vi "Save.vi"(7 "source paths":path[](array[path]), 8 "error in":errorcluster, 10 "processed sources":refnum<class "AB_Source.lvclass">[](array[class]), 11 "AB_Build in":refnum<class "AB_Build.lvclass">) -> (0 "error out":errorcluster, 1 "TypeInfo":string, 2 "source destination paths":path[](array[path]), 3 "AB_Build out":refnum<class "AB_Build.lvclass">, 4 "eng_LEIFBuildData":u32, 5 "checksums":string[](array[string]))   [LabVIEW 2020, in "AB_Build.lvclass"]
uses:
  <vilib>/AppBuilder/AB_Classes/Build/AB_Build.lvclass
  <vilib>/AppBuilder/AB_Classes/Source/AB_Source.lvclass
  <vilib>/AppBuilder/AB_Classes/Build/AB_Build.lvclass/AB_Build.ctl
  <vilib>/AppBuilder/AB_Classes/Source/VI/AB_Source_VI.lvclass
  <resource>/Framework/Providers/Common/provcom_StringGlobals.vi
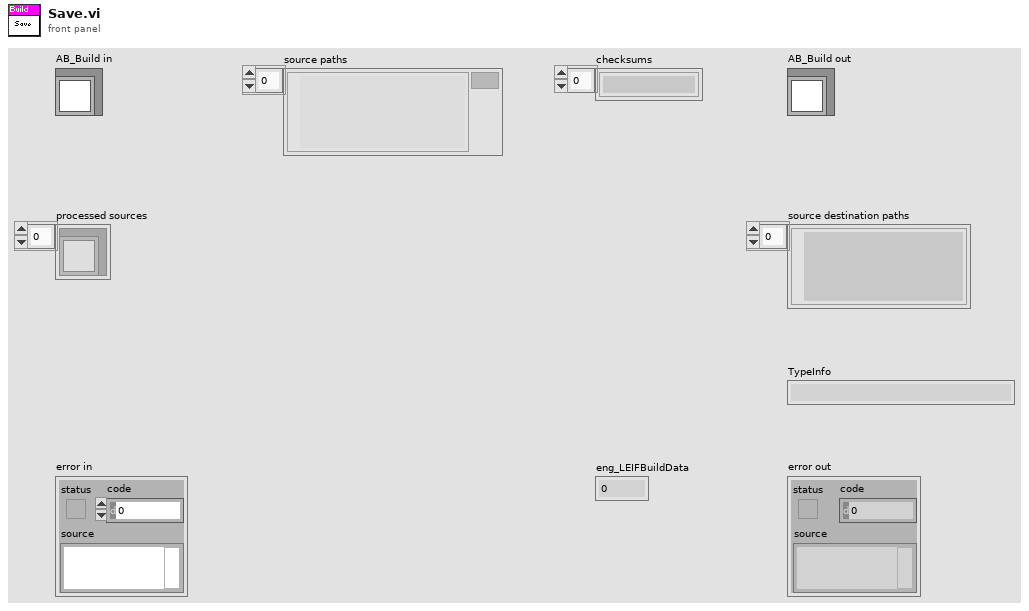
[diagram p1: front panel]
types:
  T1 = typedef "provcom_ProgressBar_Events.ctl" = cluster{"newJob":refnum<user-event>, "newItem":refnum<user-event>, "errorMsg":T2, "cancel":refnum<user-event>}
  T2 = typedef "mxLvBuildError.ctl" = refnum<user-event>
  T3 = typedef "AB_Source_Processed_Info.ctl" = cluster{"destPath":path, "buildDelimitedName":string, "sourceIndex":i32, "topLevel":bool}
  T4 = typedef "AB_Source_VI.ctl" = cluster{"standardVI":bool, "dynamicDispatch":bool, "LLBtopLevel":bool, "privateDataControl":bool, "eng_hasNonVILinks":bool, "eng_reference":refnum<vi>, "eng_saveLevel":u32}
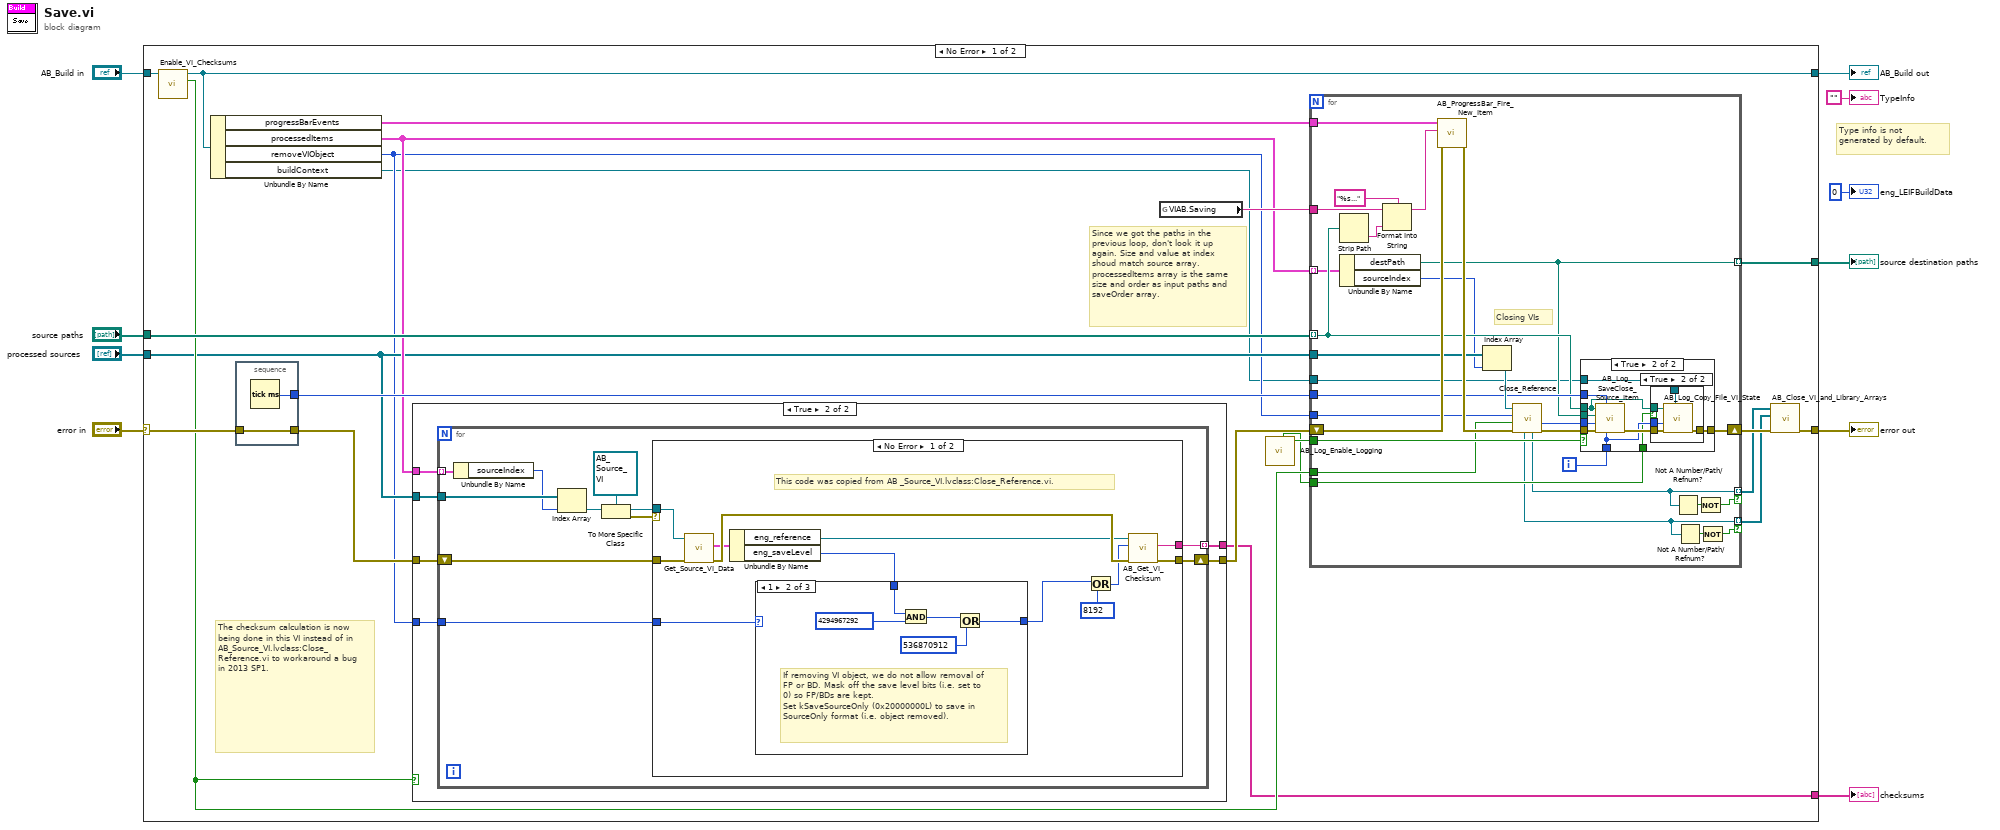
[diagram p0: block diagram]
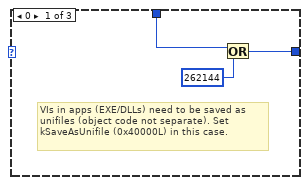
[diagram p3: hidden frame]
diagram:
  # "Type info is not generated by default."
  n1 = case shown="No Error" "error in" {
    selector: "error in" -> [w32 w122]
    tunnel: [w28 w122] -> w9
    tunnel: [w20 w121] -> w7
    tunnel: "AB_Build in" -> [w21 w121]
    tunnel: [w24 _] -> w6
    tunnel: "source paths" -> [w23 _]
    tunnel: "processed sources" -> [w17 _]
    tunnel: [w15 _] -> w2
    frame No Error {
      # "The checksum calculation is now being done in this VI instead of in AB_Source_VI.lvclass:Close_Reference.vi to workaround a bug in 2013 SP1."
      # "Since we got the paths in the previous loop, don't look it up again. Size and value at index shoud match source array. processedItems array is the same size and order as input paths and saveOrder array."
      n2 = call-dynamic "Enable_VI_Checksums.vi"("AB_Build in"=w21) -> ("VI checksums enabled?"=w19:bool, "AB_Build out"=w20:refnum<class "AB_Build.lvclass">)  [unwired: 8 in, 1 out]
      n3 = Unbundle By Name(w20) -> ("progressBarEvents"=w26:T1, "processedItems"=w18:T3[], "removeVIObject"=w16:u16, "buildContext"=w13:refnum<vi>)
      n4 = stacked-sequence {
        tunnel: w32 -> [w74]
        tunnel: [w74] -> w31
        tunnel: [w73] -> w22
        frame #0 {
          n5 = Tick Count (ms)() -> (millisecond timer value=w73:u32)
        }
      }
      n6 = case shown="True" w19 {
        tunnel: w31 -> [w33 w39]
        tunnel: [w33 w38] -> w30
        tunnel: w18 -> [_ w37]
        tunnel: w17 -> [_ w36]
        tunnel: [_ w35] -> w15
        tunnel: w16 -> [_ w34]
        frame False {
          # "Don't calculate checksums."
        }
        frame True {
          n7 = for {
            shift-right: [w48] -> w38
            shift-left: w39 -> [w49]
            tunnel: w37 -> [w47] mode=indexing
            tunnel: w36 -> [w46]
            tunnel: [w41] -> w35 mode=indexing
            tunnel: w34 -> [w40]
            n8 = Unbundle By Name(w47) -> ("sourceIndex"=w45:i32)
            n9 = Index Array(array=w46, index=w45) -> (element=w44:refnum<class "AB_Source.lvclass">)
            n10 = To More Specific Class(target class=refnum<class "AB_Source_VI.lvclass"> refnum ("AB_Source_VI.lvclass"), reference=w44) -> (specific class reference=w42:refnum<class "AB_Source_VI.lvclass">, error out=w50:errorcluster)  [unwired: 1 in]
            n11 = case shown="No Error" w50 {
              tunnel: w42 -> [w59 _]
              tunnel: w49 -> [w62 w72]
              tunnel: [w61 w72] -> w48
              tunnel: [w52 _] -> w41
              tunnel: w40 -> [w51 _]
              frame No Error {
                # "This code was copied from AB _Source_VI.lvclass:Close_Reference.vi."
                n12 = call <vilib>:"Get_Source_VI_Data.vi"("error in (no error)"=w62, "Class in"=w59) -> ("error out"=w60:errorcluster, "data"=w58:T4)  [unwired: 7 in, 1 out]
                n13 = Unbundle By Name(w58) -> ("eng_reference"=w57:refnum<vi>, "eng_saveLevel"=w54:u32)
                n14 = case shown="1" w51 {
                  tunnel: w54 -> [w65 w70 w71]
                  tunnel: [w64 w67 w71] -> w53
                  frame 0 {
                    # "VIs in apps (EXE/DLLs) need to be saved as unifiles (object code not separate). Set kSaveAsUnifile (0x40000L) in this case."
                    n15 = Or(x=w65, y=u32 262144 ("data.eng_saveLevel")) -> (x .or. y?=w64:u32)
                  }
                  frame 1 {
                    # "If removing VI object, we do not allow removal of FP or BD. Mask off the save level bits (i.e. set to 0) so FP/BDs are kept.\nSet kSaveSourceOnly (0x20000000L) to save in SourceOnly format (i.e. object removed)."
                    n16 = And(x=w70, y=u32 4294967292 ("data.eng_saveLevel")) -> (x .and. y?=w68:u32)
                    n17 = Or(x=w68, y=u32 536870912 ("data.eng_saveLevel")) -> (x .or. y?=w67:u32)
                  }
                  frame Default {
                  }
                }
                n18 = Or(x=w53, y=u32 8192 ("data.eng_saveLevel")) -> (x .or. y?=w55:u32)
                n19 = call <vilib>:"AB_Get_VI_Checksum.vi"("error in (no error)"=w60, "save level"=w55, "vi reference"=w57) -> ("error out"=w61:errorcluster, "checksum"=w52:string)  [unwired: 6 in, 1 out]
              }
              frame Error {
                # "No checksum info for non-VI types"
              }
            }
          }
        }
      }
      n20 = global read "provcom_StringGlobals.vi" "VIAB.Saving"() -> (w27:string)
      n21 = call <vilib>:"AB_Log_Enable_Logging.vi"() -> ("log?"=w25:bool, "check VI state during copy"=w14:bool)  [unwired: 2 in, 8 out]
      n22 = for {
        tunnel: w17 -> [w99]
        shift-right: [w103] -> w29
        shift-left: w30 -> [w100]
        tunnel: w25 -> [w97]
        tunnel: w26 -> [w96]
        tunnel: w27 -> [w92]
        tunnel: w23 -> [w89] mode=indexing
        tunnel: w22 -> [w90]
        tunnel: [w86] -> w24 mode=indexing
        tunnel: w18 -> [w87] mode=indexing
        tunnel: w16 -> [w84]
        tunnel: w19 -> [w83]
        tunnel: w14 -> [w82]
        tunnel: w13 -> [w81]
        tunnel: [w80] -> w11 mode=indexing if=w78
        tunnel: [w76] -> w12 mode=indexing if=w75
        i -> [w98]
        # "Closing VIs"
        n23 = Strip Path(path=w89) -> (name=w95:string)  [unwired: 1 out]
        n24 = Unbundle By Name(w87) -> ("destPath"=w86:path, "sourceIndex"=w85:i32)
        n25 = Format Into String(format string="%s..." ("initial string"), initial string=w92, w95) -> (resulting string=w94:string)  [unwired: 1 in, 1 out]
        n26 = call <vilib>:"AB_ProgressBar_Fire_New_Item.vi"("error in (no error)"=w100, "Label"=w94, "progressBarEvents in"=w96) -> ("error out"=w101:errorcluster)  [unwired: 8 out]
        n27 = Index Array(array=w99, index=w85) -> (element=w93:refnum<class "AB_Source.lvclass">)
        n28 = call-dynamic "Close_Reference.vi"("error in"=w101, "enable VI checksums"=w83, "remove VI object"=w84, "AB_Source in"=w93) -> ("error out"=w102:errorcluster, "saveLevel"=w88:u32, "Library"=w80:refnum<vi>, "VI"=w76:refnum<vi>)  [unwired: 4 out]
        n29 = case shown="True" w97 {
          tunnel: [w104 w112] -> w103
          tunnel: w98 -> [_ w108]
          tunnel: w89 -> [_ w107]
          tunnel: w102 -> [w104 w114]
          tunnel: w90 -> [_ w111]
          tunnel: w86 -> [_ w110]
          tunnel: w88 -> [_ w109]
          tunnel: w82 -> [_ w106]
          tunnel: w81 -> [_ w105]
          frame False {
          }
          frame True {
            n30 = call <vilib>:"AB_Log_SaveClose_Source_Item.vi"("index"=w108, "initial time"=w111, "error in (no error)"=w114, "saveLevel"=w109, "destinationPath"=w110, "sourcePath"=w107) -> ("error out"=w113:errorcluster)  [unwired: 5 out]
            n31 = case shown="True" w106 {
              tunnel: w113 -> [w115 w120]
              tunnel: [w115 w119] -> w112
              tunnel: w108 -> [_ w118]
              tunnel: w107 -> [_ w117]
              tunnel: w105 -> [_ w116]
              frame False {
              }
              frame True {
                n32 = call <vilib>:"AB_Log_Copy_File_VI_State.vi"("buildContext"=w116, "error in (no error)"=w120, "iteration"=w118, "sourcePath"=w117) -> ("error out"=w119:errorcluster)  [unwired: 7 out]
              }
            }
          }
        }
        n33 = Not A Number/Path/Refnum?(number/path/refnum=w80) -> (NaN/Path/Refnum?=w79:bool)
        n34 = Not A Number/Path/Refnum?(number/path/refnum=w76) -> (NaN/Path/Refnum?=w77:bool)
        n35 = Not(x=w79) -> (.not. x?=w78:bool)
        n36 = Not(x=w77) -> (.not. x?=w75:bool)
      }
      n37 = call <vilib>:"AB_Close_VI_and_Library_Arrays.vi"("error in"=w29, "VIs"=w12, "Libraries"=w11) -> ("error out"=w28:errorcluster)  [unwired: 8 in]
    }
    frame Error {
    }
  }
  "error out" <- w9
  "AB_Build out" <- w7
  "source destination paths" <- w6
  "checksums" <- w2
  "TypeInfo" <- ""
  "eng_LEIFBuildData" <- u32 0 ("Numeric")
